vi "ListboxGlobal.vi"() -> ()   [LabVIEW 2017]
panel:
  in  "Constant.not present":string="- not added -"
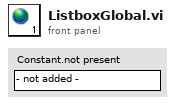
[diagram p1: front panel]
diagram:
